vi "Create Status Log File.vi"(7 "QRD":T1, 8 "error in":errorcluster) -> (0 "error out":errorcluster, 5 "QRD Out":T1)   [LabVIEW 2025]
uses:
  Controls/Queues-Refs-Data.ctl
  Builds/Queue Wrappers.lvlibp/Q Packet.ctl
  Libraries/File-Utilities/File Utilities.lvlibp
  Builds/Queue Wrappers.lvlibp
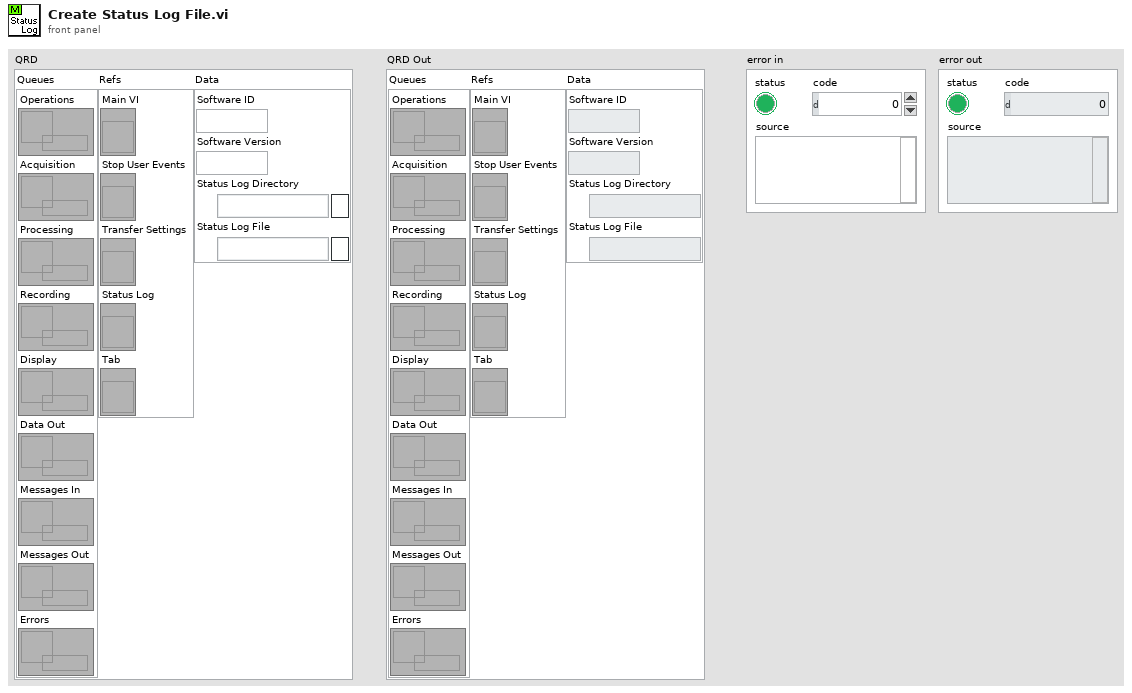
[diagram p1: front panel]
types:
  T1 = typedef "Queues-Refs-Data.ctl" = cluster{"Queues":cluster{"Operations":refnum<queue>, "Acquisition":refnum<queue>, "Processing":refnum<queue>, "Recording":refnum<queue>, "Display":refnum<queue>, "Data Out":refnum<queue>, "Messages In":refnum<queue>, "Messages Out":refnum<queue>, "Errors":refnum<queue>}, "Refs":cluster{"Main VI":refnum<vi>, "Stop User Events":refnum<vi>, "Transfer Settings":refnum<vi>, "Status Log":refnum<vi>, "Tab":refnum<vi>}, "Data":cluster{"Software ID":string, "Software Version":string, "Status Log Directory":path, "Status Log File":path}}
  T2 = enum16{"open", "replace", "create", "open or create", "replace or create", "replace or create with confirmation"}
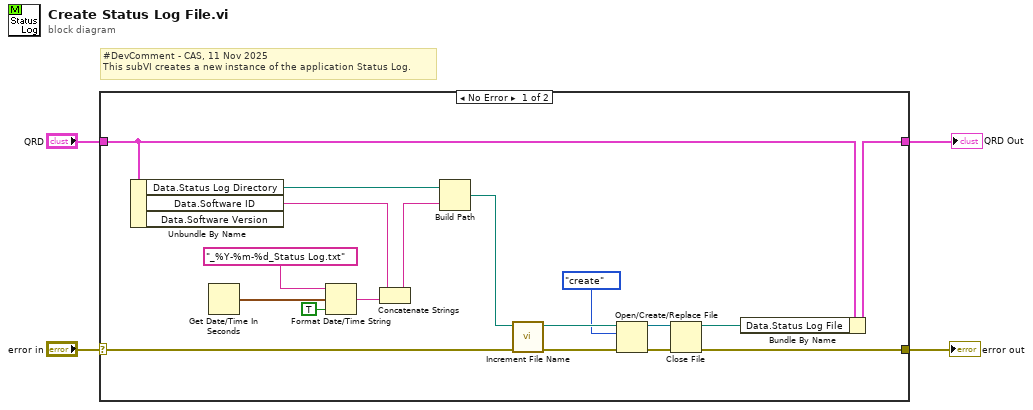
[diagram p0: block diagram]
diagram:
  # "#DevComment - CAS, 11 Nov 2025\nThis subVI creates a new instance of the application Status Log."
  n1 = case shown="No Error" "error in" {
    selector: "error in" -> [w15 w24]
    tunnel: "QRD" -> [w12 w23]
    tunnel: [w8 w24] -> w2
    tunnel: [w13 w23] -> w1
    frame No Error {
      n2 = Unbundle By Name(w12) -> ("Data.Status Log Directory"=w22:path, "Data.Software ID"=w21:string)  [unwired: 1 out]
      n3 = Get Date/Time In Seconds() -> (seconds since 1Jan1904=w19:timestamp)
      n4 = Format Date/Time String(time format string (%c)="_%Y-%m-%d_Status Log.txt", seconds (now)=w19, UTC format=TRUE) -> (date/time string=w16:string)
      n5 = Concatenate Strings(w21, w16) -> (w20:string)
      n6 = Build Path(base path=w22, name or relative path=w20) -> (appended path=w14:path)
      n7 = call "Increment File Name.vi"("error in"=w15, "File Path"=w14) -> ("error out"=w10:errorcluster, "File Path Out"=w11:path)  [unwired: 8 in]
      n8 = Open/Create/Replace File(file path (use dialog)=w11, error in=w10, operation (0:open)=T2."create") -> (refnum out=w7:refnum<file>, error out=w9:errorcluster)  [unwired: 3 in, 1 out]
      n9 = Close File(refnum=w7, error in=w9) -> (path=w6:path, error out=w8:errorcluster)
      n10 = Bundle By Name(cluster=w12, "Data.Status Log File"=w6) -> (w13:T1)
    }
    frame Error {
    }
  }
  "QRD Out" <- w1
  "error out" <- w2
